vi "Get (U16).vi"(8 "error in":errorcluster, 11 "Value in":refnum<class "Value.lvclass">) -> (0 "error out":errorcluster, 1 "Defined?":bool, 2 "Value":u16, 3 "Value out":refnum<class "Value.lvclass">)   [LabVIEW 2024, in "EDS.lvlib" / "Value.lvclass"]
uses:
  Value.lvclass
  Value.lvclass/Value.ctl
  EDS.lvlib
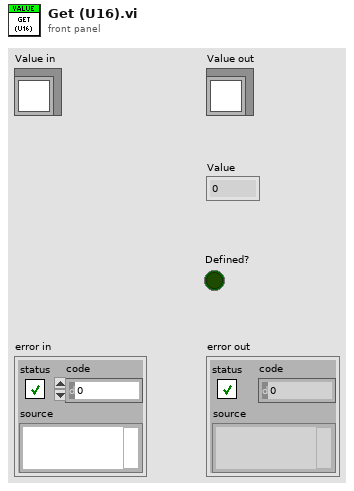
[diagram p1: front panel]
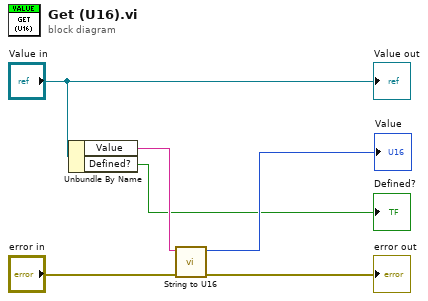
[diagram p0: block diagram]
diagram:
  n1 = Unbundle By Name("Value in") -> ("Value"=w5:string, "Defined?"=→"Defined?":bool)
  n2 = call "String to U16.vi"("error in"="error in", "String"=w5) -> ("error out"=→"error out":errorcluster, "U16"=→"Value":u16)  [unwired: 8 in]
  "Value out" <- "Value in"
